vi "fpga_W&R_ADC_Write_then_CLK.vi"() -> ()   [LabVIEW 2018]
uses:
  <vilib>/rvi/Emulation/niFpgaGetClockAttributes.vi
  <vilib>/rvi/Emulation/niFpgaSctlEmulationGetInTimedLoop.vi
  <vilib>/rvi/Emulation/niFpgaEmulationReportErrorSimple.vi
  <vilib>/rvi/eio/common/nirviEmuTemplateMethod_errors.vi
  <vilib>/rvi/Emulation/niFpgaCriticalErrorInLSC.vi
  <vilib>/eio/EIONode/EIONode.xnode
panel:
  out "ADC read":bool[](array[boolean])=[FALSE, FALSE, FALSE, TRUE, TRUE, TRUE, FALSE, TRUE, FALSE, TRUE, FALSE, FALSE, FALSE, TRUE, FALSE, FALSE]
  in  "ADC write":bool[](array[boolean])=[FALSE, FALSE, FALSE, FALSE, FALSE, TRUE, FALSE, FALSE, FALSE, FALSE, FALSE, FALSE, FALSE, FALSE, FALSE, FALSE]
  in  "delay (us)":u32=40000
  in  "Stop":bool
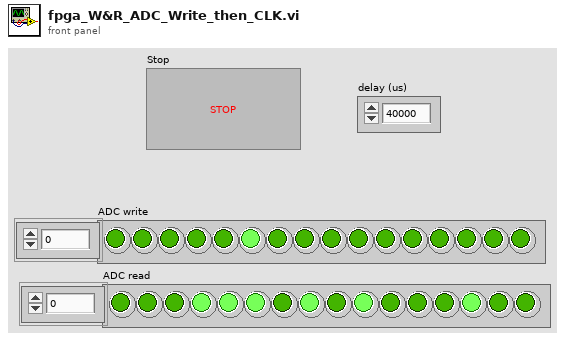
[diagram p1: front panel]
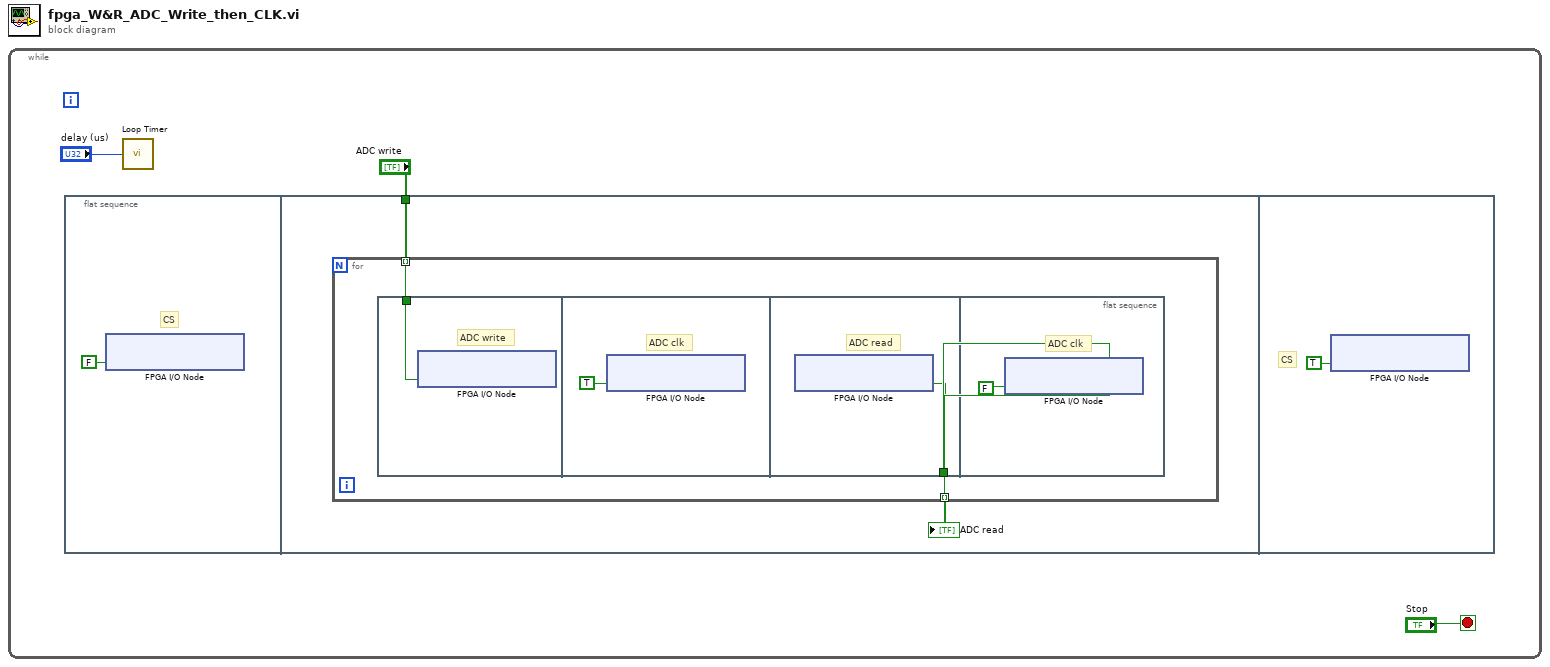
[diagram p0: block diagram]
diagram:
  n1 = while {
    stop <- "Stop" stop-if-true
    n2 = flat-sequence {
      tunnel: "ADC write" -> [w6]
      frame #0 {
        # "CS"
        n3 = xnode "FPGA I/O Node"("ConnectorA/DIO4"=FALSE) -> ()  [unwired: 1 in, 1 out]
      }
      frame #1 {
        n4 = for {
          tunnel: w6 -> [w8] mode=indexing
          tunnel: [w7] -> w5 mode=indexing
          n5 = flat-sequence {
            tunnel: w8 -> [w9]
            tunnel: [w11] -> w7
            frame #0 {
              # "ADC write"
              n6 = xnode "FPGA I/O Node"("ConnectorA/DIO2"=w9) -> ()  [unwired: 1 in, 1 out]
            }
            frame #1 {
              # "ADC clk"
              n7 = xnode "FPGA I/O Node"("ConnectorA/DIO3"=TRUE) -> ()  [unwired: 1 in, 1 out]
            }
            frame #2 {
              # "ADC read"
              n8 = xnode "FPGA I/O Node"() -> ("ConnectorA/DIO1"=w11:bool)  [unwired: 1 in, 1 out]
            }
            frame #3 {
              # "ADC clk"
              n9 = xnode "FPGA I/O Node"("ConnectorA/DIO3"=FALSE) -> ()  [unwired: 1 in, 1 out]
            }
          }
        }
        "ADC read" <- w5
      }
      frame #2 {
        # "CS"
        n10 = xnode "FPGA I/O Node"("ConnectorA/DIO4"=TRUE) -> ()  [unwired: 1 in, 1 out]
      }
    }
    n11 = call "Loop Timer"("Count(Ticks)"="delay (us)") -> ()  [unwired: 1 out]
  }
